vi "ReadStringIniKey.vi"(8 "error in (no error)":errorcluster, 9 "Key":string, 10 "Section":string, 11 "refnum In":T1) -> (0 "error out":errorcluster, 2 "Value":string, 3 "refnum out":T1)   [LabVIEW 2013]
uses:
  <vilib>/Utility/config.llb/Config Data RefNum.ctl
  090 - ERRORS/Ctrls/EnumErrors.ctl
  <vilib>/Utility/config.llb/Read Key (String).vi
  <vilib>/Utility/config.llb/NI_LVConfig.lvlib
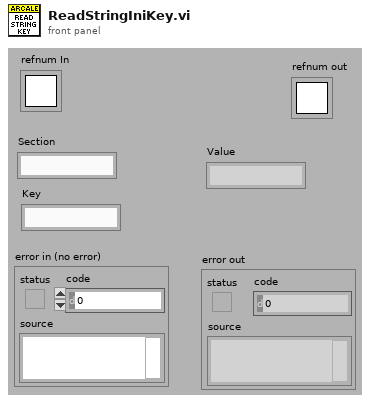
[diagram p1: front panel]
types:
  T1 = typedef "NI_LVConfig.lvlib/Config Data RefNum.ctl" = refnum<k1>
  T2 = typedef "EnumErrors.ctl" = enum16{"VI non trouvé !", "Clé non trouvée", "Timeout", "Le VI tourne déjà", "Erreur de séparateur décimal", "Référence non trouvée"}
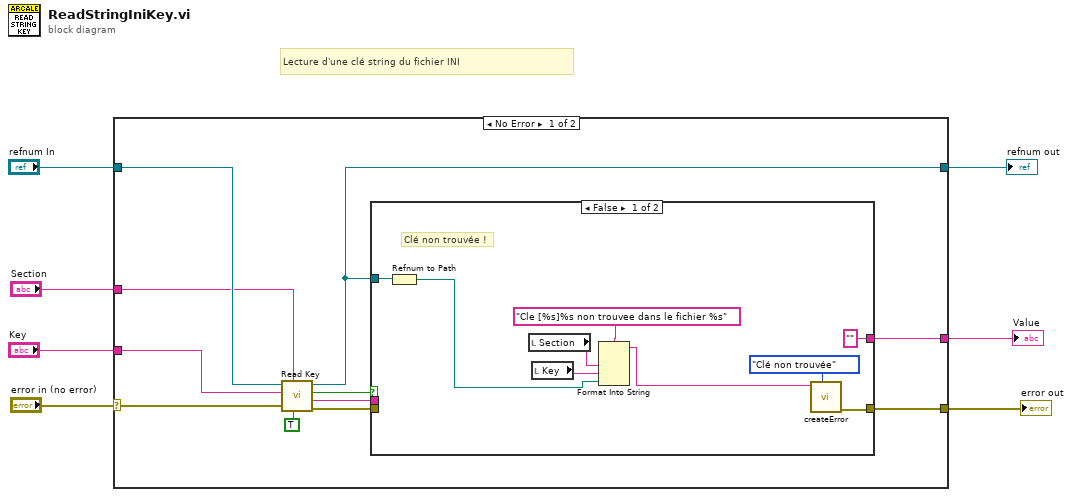
[diagram p0: block diagram]
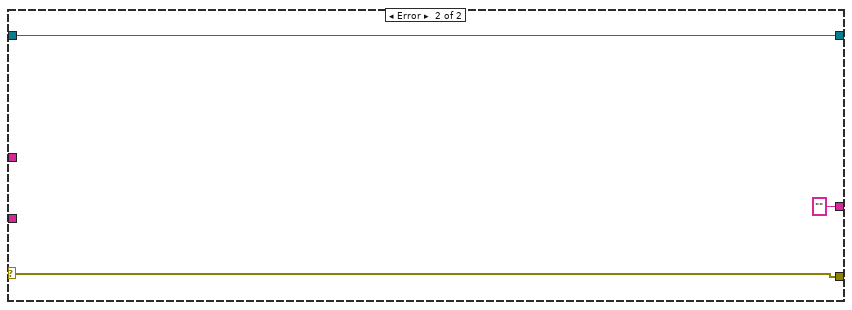
[diagram p3: hidden frame]
diagram:
  # "Lecture d'une clé string du fichier INI"
  n1 = case shown="No Error" "error in (no error)" {
    selector: "error in (no error)" -> [w18 w32]
    tunnel: "refnum In" -> [w17 w30]
    tunnel: "Section" -> [w16 _]
    tunnel: "Key" -> [w15 _]
    tunnel: [w8 w30] -> w3
    tunnel: [w10 "" ("value")] -> w2
    tunnel: [w9 w32] -> w1
    frame No Error {
      n2 = call-poly <vilib>:"Read Key.vi"("read raw string? (F)"=TRUE, "section"=w16, "error in (no error)"=w18, "key"=w15, "refnum"=w17) -> ("error out"=w12:errorcluster, "value"=w11:string, "found?"=w13:bool, "refnum out"=w8:T1)  [unwired: 1 in, 2 out]
      n3 = case shown="False" w13 {
        tunnel: w12 -> [_ w29]
        tunnel: w11 -> [_ w28]
        tunnel: ["" ("value") w28] -> w10
        tunnel: [w23 w29] -> w9
        tunnel: w8 -> [w21 _]
        frame False {
          # "Clé non trouvée !"
          n4 = Refnum to Path(1:w21) -> (0:w20:path)
          n5 = local read "Section"() -> (w26:string)
          n6 = local read "Key"() -> (w25:string)
          n7 = Format Into String(format string="Cle [%s]%s non trouvee dans le fichier %s", w26, w25, w20) -> (resulting string=w22:string)  [unwired: 2 in, 1 out]
          n8 = call "createError.vi"("ErrorCode"=EnumErrors."Clé non trouvée", "message"=w22) -> ("error out"=w23:errorcluster)  [unwired: 2 in, 7 out]
        }
        frame True {
          # "Clé trouvée !!!"
        }
      }
    }
    frame Error {
    }
  }
  "error out" <- w1
  "refnum out" <- w3
  "Value" <- w2
